vi "Set Driver Controls.vi"(4 "Background Image":refnum<vi>, 5 "Abort":refnum<vi>, 6 "Inkscape File (.svg)":refnum<vi>, 7 "Run":refnum<vi>, 8 "error in (no error)":errorcluster, 9 "Data Queue":refnum<queue>, 10 "Lithography Data":T2(array[cluster]), 11 "VI in":refnum<vi>) -> (0 "error out":errorcluster, 3 "VI out":refnum<vi>)   [LabVIEW 2020]
uses:
  <userlib>/LevyLab/Relay Box/Type_defs/Resistor--enum.ctl
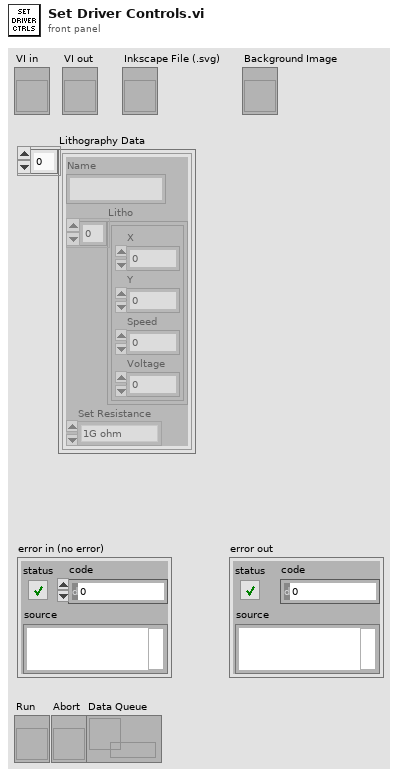
[diagram p1: front panel]
types:
  T1 = typedef "Resistor--enum.ctl" = enum16{"open", "discharge tip", "0 ohms", "100k ohm", "10M ohm", "1G ohm"}
  T2 = cluster{"Name":string, "Litho":cluster{"X":dbl, "Y":dbl, "Speed":dbl, "Voltage":dbl}[], "Set Resistance":T1}[]
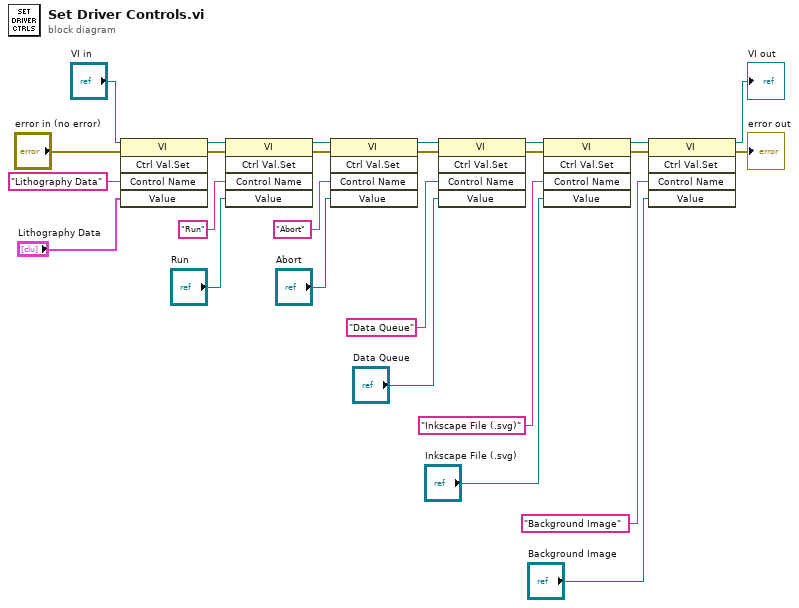
[diagram p0: block diagram]
diagram:
  n1 = invoke class="VI" method="Ctrl Val.Set"(reference="VI in", error in="error in (no error)", "Control Name"="Lithography Data", "Value"="Lithography Data") -> (reference out=w20:refnum<vi>, error out=w19:errorcluster)  [unwired: 1 in, 3 out]
  n2 = invoke class="VI" method="Ctrl Val.Set"(reference=w20, error in=w19, "Control Name"="Run", "Value"="Run") -> (reference out=w22:refnum<vi>, error out=w21:errorcluster)  [unwired: 1 in, 3 out]
  n3 = invoke class="VI" method="Ctrl Val.Set"(reference=w22, error in=w21, "Control Name"="Abort", "Value"="Abort") -> (reference out=w14:refnum<vi>, error out=w13:errorcluster)  [unwired: 1 in, 3 out]
  n4 = invoke class="VI" method="Ctrl Val.Set"(reference=w14, error in=w13, "Control Name"="Data Queue", "Value"="Data Queue") -> (reference out=w11:refnum<vi>, error out=w10:errorcluster)  [unwired: 1 in, 3 out]
  n5 = invoke class="VI" method="Ctrl Val.Set"(reference=w11, error in=w10, "Control Name"="Inkscape File (.svg)", "Value"="Inkscape File (.svg)") -> (reference out=w9:refnum<vi>, error out=w8:errorcluster)  [unwired: 1 in, 3 out]
  n6 = invoke class="VI" method="Ctrl Val.Set"(reference=w9, error in=w8, "Control Name"="Background Image", "Value"="Background Image") -> (reference out=→"VI out":refnum<vi>, error out=→"error out":errorcluster)  [unwired: 1 in, 3 out]
